vi "Joystick Mapping Function.vi"(10 "Gain":dbl, 11 "Dead Zone":i32) -> (3 "Gain Out":dbl)   [LabVIEW 2014]
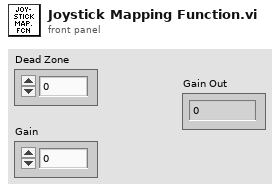
[diagram p1: front panel]
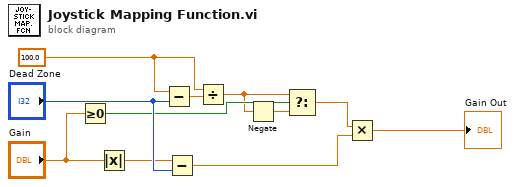
[diagram p0: block diagram]
diagram:
  w11 = 100.0
  n1 = Greater Or Equal To 0?(x="Gain") -> (x >= 0?=w5:bool)
  n2 = Absolute Value(x="Gain") -> (abs(x)=w1:dbl)
  n3 = Subtract(x=w11, y="Dead Zone") -> (x-y=w8:dbl)
  n4 = Subtract(x=w1, y="Dead Zone") -> (x-y=w7:dbl)
  n5 = Divide(x=w11, y=w8) -> (x/y=w3:dbl)
  n6 = Negate(x=w3) -> (-x=w4:dbl)
  n7 = Select(t=w3, s=w5, f=w4) -> (s? t:f=w6:dbl)
  n8 = Multiply(x=w6, y=w7) -> (x*y=→"Gain Out":dbl)
